vi "newDevice.vi"(8 "error in (no error)":errorcluster, 10 "Device Type":T1, 11 "reference in":refnum<class "Project Panels.lvclass">=refnum) -> (0 "error out":errorcluster={"status"=TRUE, "code"=1556, "source"="In Place Element Structure in File Controller.lvclass:getExcelFileRefs.vi->Devices Controller.lvclass:newDevice.vi->Project Panels.lvclass:newItem.vi->Project Panels.lvclass:products.vi->GUI Controller.lvclass:operate.vi->Master Controller.lvclass:operate.vi->main.vi"}, 2 "saved?":bool, 3 "reference out":refnum<class "Project Panels.lvclass">)   [LabVIEW 2016, in "Project Panels.lvclass"]
uses:
  Project Panels.lvclass
  SYS/Devices Controller_llb/deviceType.ctl
  deviceState.ctl
  SYS/Devices Controller_llb/Devices Controller.lvclass
panel:
  out "title":string="New ...."
  in  "City":string
  in  "End User Email":string
  in  "End User":string
  in  "System's Location":string
  in  "Account":string
  in  "Description":string
  in  "SW Version":string
  in  "S/N":string
  out "statusBar":string
  in  "Save Button":bool
  in  "Stop Button":bool
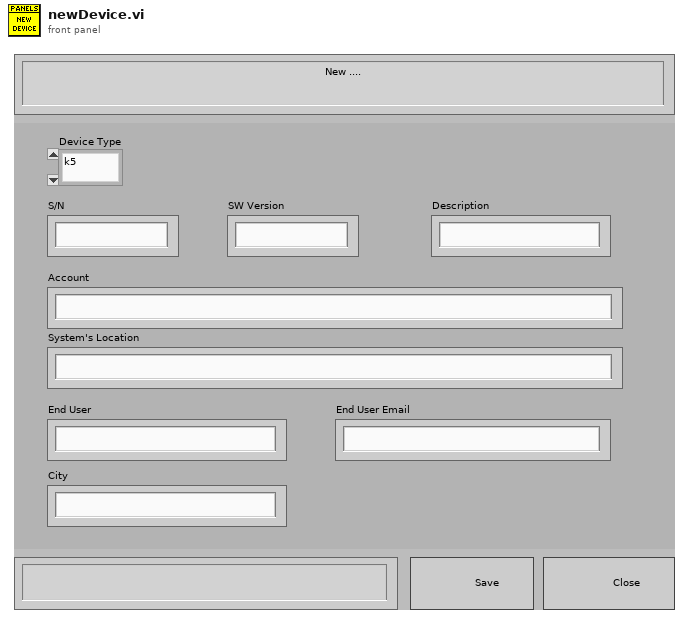
[diagram p1: front panel]
types:
  T1 = typedef "Devices Controller.lvclass/deviceType.ctl" = enum16{"k5", "k4b2", "fitmate", "cpet", "rmr", "bodyBoxPft", "bp", "pp"}
  T2 = cluster{"deviceType":T1, "S/N":string, "SW":string, "Description":string, "Account":string, "System's Location":string, "End User":string, "Email":string, "City":string, "FollowUp Sent":string, "FollowUp Accepted":string}
  T3 = typedef "Project Panels.lvclass/deviceState.ctl" = enum16{"check", "initiate", "waitEvent", "dataFromPDF", "getDetails", "TSR", "save", "close", "stop"}
  T4 = cluster{"deviceType":T1, "S/N":string, "SW":string, "Description":string, "Account":string, "System's Location":string, "End User":string, "Email":string, "City":string, "LastChange":string, "Service By":string, "Exp Date":string, "FollowUp Sent":string, "FollowUp Accepted":string, "Note":string}
  T5 = typedef "Project Panels.lvclass/ObjectAttributesRef.ctl" = refnum<data-value>
  T6 = typedef "Project Panels.lvclass/ObjectAttributes.ctl" = cluster{"MyAttribute":dbl, "device_controller_ref":refnum<class "Devices Controller.lvclass">, "file_controller_ref":refnum<class "File Controller.lvclass">, "item_controller_ref":refnum<class "Items Controller.lvclass">, "item_tables":cluster{"checkIN":string[][], "checkOUT":string[][], "storage":string[][]}, "quickbook_table":cluster{"notes":string[][]}, "notification_controller_ref":refnum<class "Notification Controller.lvclass">, "partstracking_controller_ref":refnum<class "PartsTracking Controller.lvclass">, "product_tables":cluster{"k4b2":string[][], "fitmate":string[][], "RMR":string[][], "CPET":string[][], "BP":string[][], "PP":string[][], "k5":string[][], "bb-pft":string[][]}, "rowsColour":u32[], "low_resolution?":bool, "run_python?":bool}
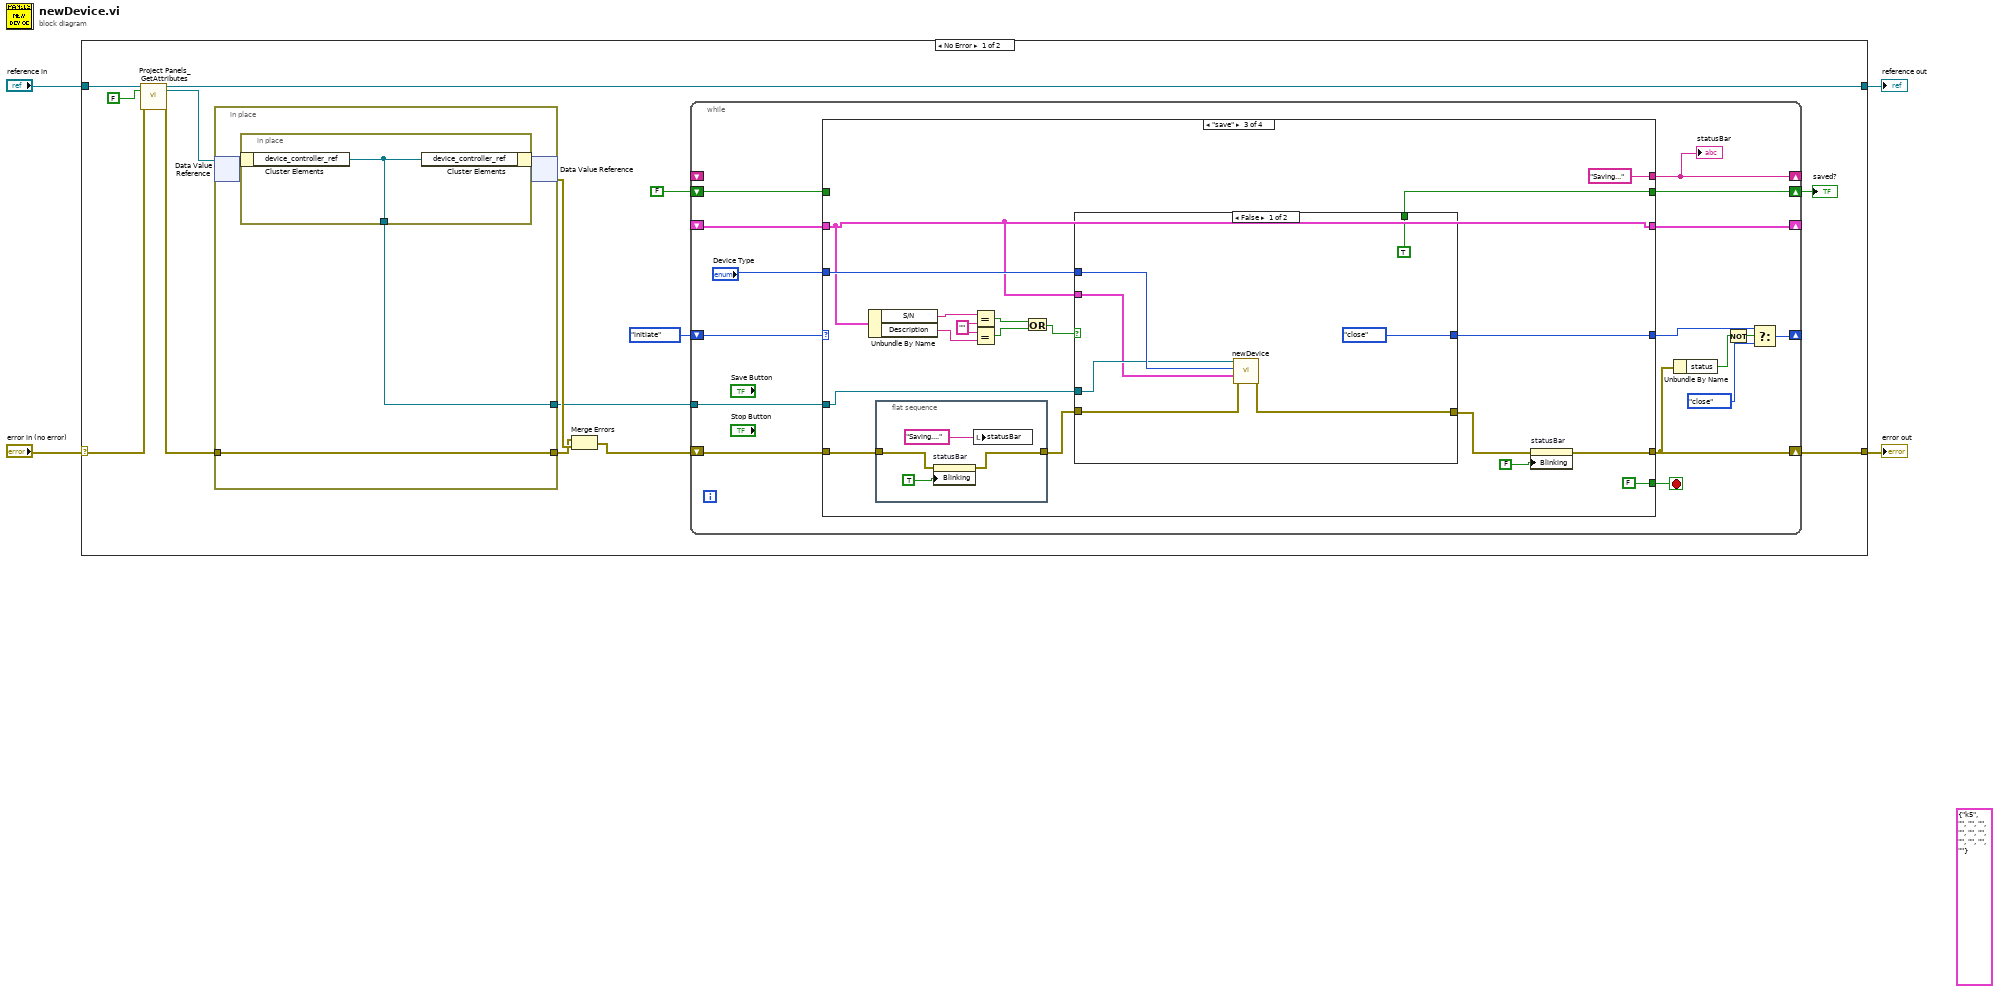
[diagram p0: block diagram]
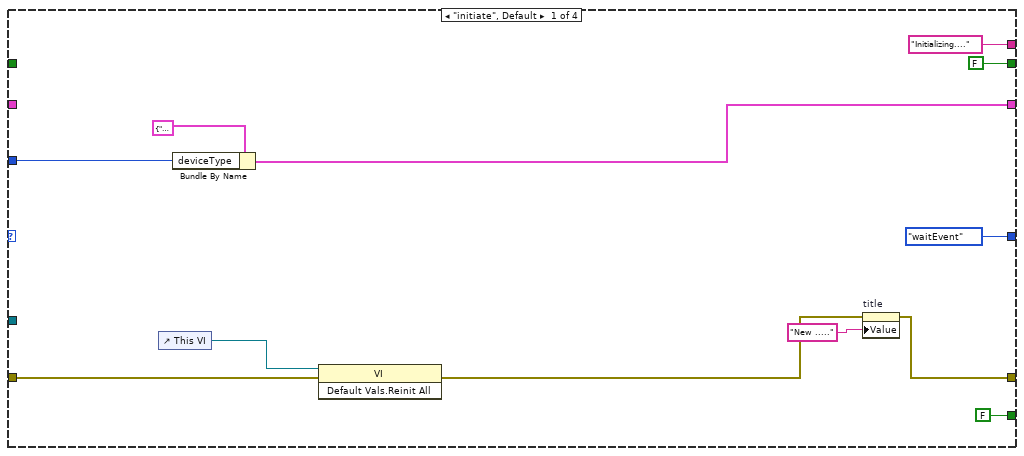
[diagram p2: hidden frame]
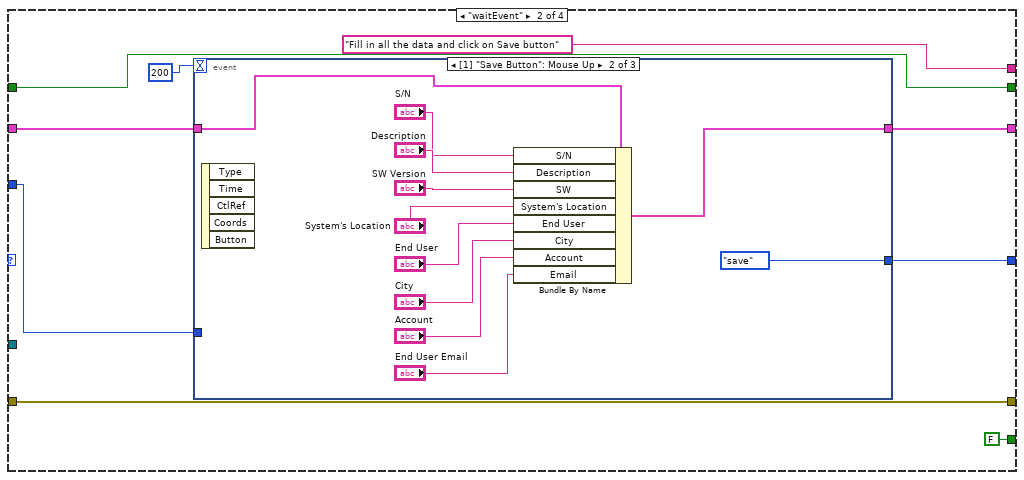
[diagram p3: hidden frame]
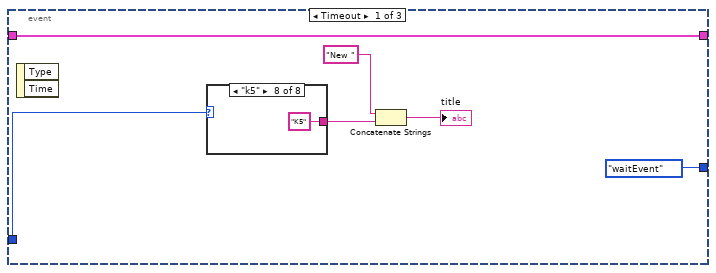
[diagram p4: hidden frame]
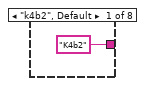
[diagram p5: hidden frame]
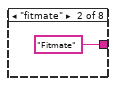
[diagram p6: hidden frame]
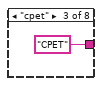
[diagram p7: hidden frame]
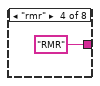
[diagram p8: hidden frame]
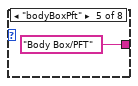
[diagram p9: hidden frame]
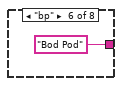
[diagram p10: hidden frame]
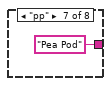
[diagram p11: hidden frame]
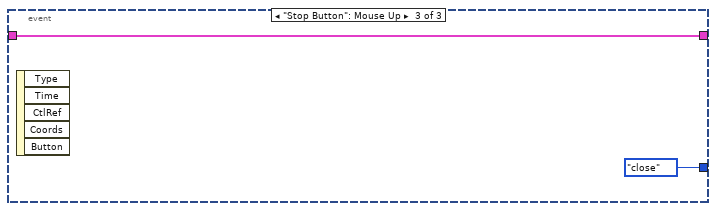
[diagram p12: hidden frame]
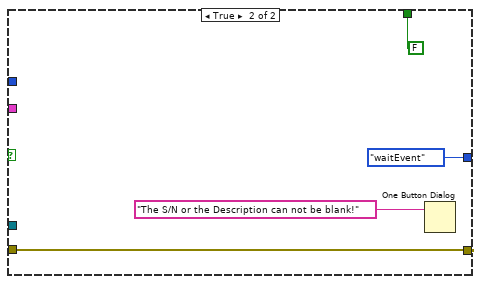
[diagram p13: hidden frame]
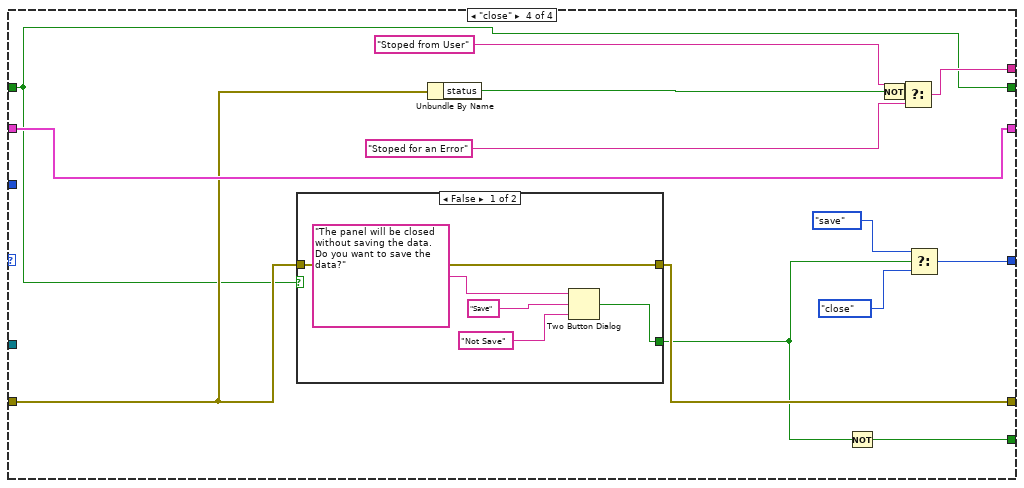
[diagram p14: hidden frame]
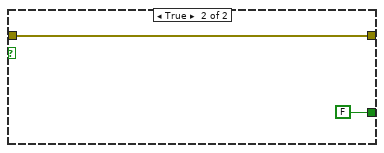
[diagram p15: hidden frame]
diagram:
  (unwired) T2 {"deviceType"=enum."k5", "S/N"="", "SW"="", "Description"="", "Account"="", "System's Location"="", "End User"="", "Email"="", "City"="", "FollowUp Sent"="", "FollowUp Accepted"=""} ("details")
  n1 = case shown="No Error" "error in (no error)" {
    selector: "error in (no error)" -> [w14 w143]
    tunnel: [w9 w143] -> w3
    tunnel: [w12 w142] -> w1
    tunnel: "reference in" -> [w16 w142]
    frame No Error {
      n2 = call "Project Panels_GetAttributes.vi"("reference in"=w16, "return data? (T)"=FALSE, "error in (no error)"=w14) -> ("reference out"=w12:refnum<class "Project Panels.lvclass">, "attributes ref"=w11:T5, "error out"=w13:errorcluster)  [unwired: 13 in, 1 out]
      n3 = in-place {
        in-place-border: w13 -> [w138]
        in-place-border: [w138] -> w17
        in-place-border: [w137] -> w7
        n4 = in-place-dvr #1(w11) -> (w139:T6)  [unwired: 1 out]
        n5 = in-place {
          in-place-border: [w141] -> w137
          n6 = in-place-cluster #2(w139) -> ("device_controller_ref"=w141:refnum<class "Devices Controller.lvclass">)
          n7 = in-place-cluster #2("device_controller_ref"=w141) -> (w140:T6)
        }
        n8 = in-place-dvr #1(w140) -> (w18:errorcluster)  [unwired: 1 out]
      }
      n9 = Merge Errors(w17, w18) -> (w10:errorcluster)
      n10 = while {
        shift-right: [w23] -> w9
        shift-left: w10 -> [w34]
        shift-right: [w24] -> _
        shift-left: deviceState."initiate" ("state") -> [w33]
        shift-right: [w31] -> _
        shift-left: _ -> [w30]
        shift-right: [w29] -> _
        shift-left: _ -> [_]
        tunnel: w7 -> [w28]
        shift-right: [w27] -> w5
        shift-left: FALSE -> [w26]
        stop <- w32 stop-if-true
        n11 = case shown="\"save\"" w33 {
          tunnel: w34 -> [w37 w55 w88 w123]
          tunnel: [w40 w55 w84 w122] -> w23
          tunnel: [FALSE FALSE FALSE w117] -> w32
          tunnel: [deviceState."waitEvent" ("state") w53 w93 w121] -> w25
          tunnel: "Device Type" -> [w43 w50 w92 _]
          tunnel: [w44 w47 w89 w125] -> w31
          tunnel: w30 -> [_ w48 w89 w125]
          tunnel: ["Initializing...." ("statusBar") "Fill in all the data and click on Save button" ("statusBar") "Saving..." ("title") w124] -> w29
          tunnel: w28 -> [_ _ w91 _]
          tunnel: [FALSE w49 w90 w116] -> w27
          tunnel: w26 -> [_ w49 _ w116]
          frame "initiate", Default {
            n12 = control-ref of="This VI"() -> (w38:refnum<vi>)
            n13 = Bundle By Name(cluster=T4 {"deviceType"=enum."k5", "S/N"="", "SW"="", "Description"="", "Account"="", "System's Location"="", "End User"="", "Email"="", "City"="", "LastChange"="", "Service By"="", "Exp Date"="", "FollowUp Sent"="", "FollowUp Accepted"="", "Note"=""} ("details"), "deviceType"=w43) -> (w44:T4)
            n14 = invoke class="VI" method="Default Vals.Reinit All"(reference=w38, error in=w37) -> (error out=w36:errorcluster)  [unwired: 1 in, 2 out]
            n15 = property on="title" class="Str"(error in=w36, "Value"="New ....." ("title")) -> (error out=w40:errorcluster)  [unwired: 1 in, 1 out]
          }
          frame "waitEvent" {
            n16 = event shown="[1] \"Save Button\": Mouse Up" {
              selector: _ -> [_ _ _]
              dyn-events: _ -> [_ _ _]
              timeout: 200 -> [_ _ _]
              tunnel: [deviceState."waitEvent" ("state") deviceState."save" ("state") deviceState."close" ("state")] -> w53
              tunnel: w50 -> [w57 _ _]
              tunnel: w48 -> [w56 w71 w81]
              tunnel: [w56 w70 w81] -> w47
              event Timeout {
                n17 = event-data() -> ()  [unwired: 1 in, 2 out]
                n18 = case shown="\"k5\"" w57 {
                  tunnel: ["K4b2" ("title") "Fitmate" ("title") "CPET" ("title") "RMR" ("title") "Body Box/PFT" ("title") "Bod Pod" ("title") "Pea Pod" ("title") "K5" ("title")] -> w59
                  frame "k4b2", Default {
                  }
                  frame "fitmate" {
                  }
                  frame "cpet" {
                  }
                  frame "rmr" {
                  }
                  frame "bodyBoxPft" {
                  }
                  frame "bp" {
                  }
                  frame "pp" {
                  }
                  frame "k5" {
                  }
                }
                n19 = Concatenate Strings("New " ("title"), w59) -> (→"title":string)
              }
              event "Save Button": Mouse Up {
                n20 = event-data() -> ()  [unwired: 1 in, 5 out]
                n21 = Bundle By Name(cluster=w71, "S/N"="S/N", "Description"="Description", "SW"="SW Version", "System's Location"="System's Location", "End User"="End User", "City"="City", "Account"="Account", "Email"="End User Email") -> (w70:T4)
              }
              event "Stop Button": Mouse Up {
                n22 = event-data() -> ()  [unwired: 1 in, 5 out]
              }
            }
          }
          frame "save" {
            w97 = "" ("y")
            n23 = Unbundle By Name(w89) -> ("S/N"=w99:string, "Description"=w98:string)
            n24 = flat-sequence {
              tunnel: [w102] -> w87
              tunnel: w88 -> [w103]
              frame #0 {
                n25 = property on="statusBar" class="Str"(error in=w103, "Blinking"=TRUE) -> (error out=w102:errorcluster)  [unwired: 1 in, 1 out]
                n26 = local write "statusBar"("Saving...." ("statusBar")) -> ()
              }
            }
            n27 = Equal?(x=w99, y=w97) -> (x = y?=w96:bool)
            n28 = Equal?(x=w97, y=w98) -> (x = y?=w95:bool)
            n29 = Or(x=w96, y=w95) -> (x .or. y?=w94:bool)
            n30 = case shown="False" w94 {
              tunnel: w87 -> [w109 w112]
              tunnel: [w105 w112] -> w85
              tunnel: [deviceState."close" ("state") deviceState."waitEvent" ("state")] -> w93
              tunnel: w92 -> [w108 _]
              tunnel: w91 -> [w107 _]
              tunnel: [TRUE FALSE] -> w90
              tunnel: w89 -> [w106 _]
              frame False {
                n31 = call "newDevice.vi"("error in (no error)"=w109, "details"=w106, "Device Type"=w108, "reference in"=w107) -> ("error out"=w105:errorcluster)  [unwired: 6 in, 1 out]
              }
              frame True {
                n32 = One Button Dialog(message="The S/N or the Description can not be blank!") -> ()  [unwired: 1 in, 1 out]
              }
            }
            n33 = property on="statusBar" class="Str"(error in=w85, "Blinking"=FALSE) -> (error out=w84:errorcluster)  [unwired: 1 in, 1 out]
          }
          frame "close" {
            n34 = case shown="False" w116 {
              tunnel: w123 -> [w134 w135]
              tunnel: [w134 w135] -> w122
              tunnel: [w132 FALSE ("Save")] -> w118
              frame False {
                n35 = Two Button Dialog(message="The panel will be closed without saving the data. Do you want to save the data?", 1:"Not Save" ("F button name (\"Cancel\")"), 2:"Save" ("T button name (\"OK\")")) -> (T button?=w132:bool)
              }
              frame True {
              }
            }
            n36 = Unbundle By Name(w123) -> ("status"=w129:bool)
            n37 = Not(x=w118) -> (.not. x?=w117:bool)
            n38 = Not(x=w129) -> (.not. x?=w126:bool)
            n39 = Select(t="Stoped from User" ("title"), s=w126, f="Stoped for an Error" ("title")) -> (s? t:f=w124:string)
            n40 = Select(t=deviceState."save" ("state"), s=w118, f=deviceState."close" ("state")) -> (s? t:f=w121:T3)
          }
        }
        "statusBar" <- w29
        n41 = Unbundle By Name(w23) -> ("status"=w22:bool)
        n42 = Not(x=w22) -> (.not. x?=w20:bool)
        n43 = Select(t=w25, s=w20, f=deviceState."close") -> (s? t:f=w24:T3)
      }
      "saved?" <- w5
    }
    frame Error {
    }
  }
  "error out" <- w3
  "reference out" <- w1
